vi "Read Persistent Unified Msgs.vi"(11 "Attributes in":refnum<class "Attributes.lvclass">) -> (2 "Persistent Unified Msgs":T1)   [LabVIEW 2025, in "jettl.lvlib" / "Attributes.lvclass"]
uses:
  Attributes.lvclass
  Msgs.ctl
  Msg/Msg.lvclass
  jettl.lvlib
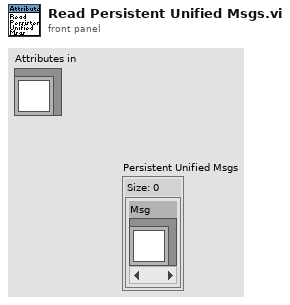
[diagram p1: front panel]
types:
  T1 = typedef "jettl.lvlib/Msgs.ctl" = set{refnum<class "Msg.lvclass">}
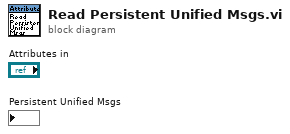
[diagram p0: block diagram]
diagram:
